vi "SetHasckelAO.vi"(0 "FPGA API in":refnum<class "FPGA API Mock.lvclass">, 5 "Haskel in":dbl, 11 "error in (no error)":errorcluster) -> (4 "FPGA API out":refnum<class "FPGA API Mock.lvclass">, 15 "error out":errorcluster)   [LabVIEW 2019, in "FPGA API Mock.lvclass"]
uses:
  FPGA API Mock.lvclass
  FPGA API Mock.lvclass/FPGA API Mock.ctl
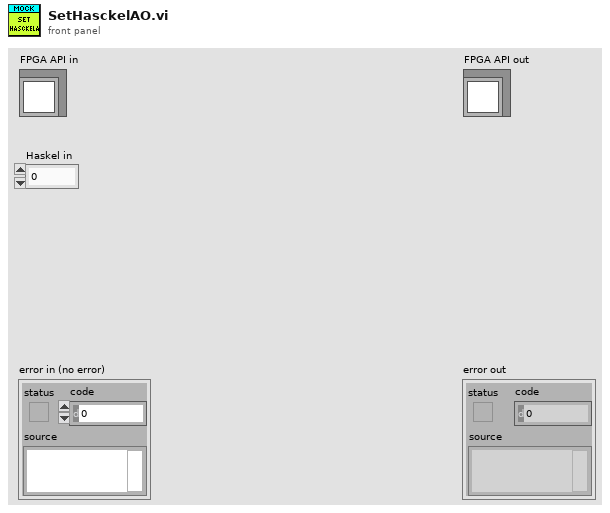
[diagram p1: front panel]
types:
  T1 = typedef "FPGA API Mock.lvclass/Data.ctl" = cluster{"DO":bool[], "DI":bool[], "AI":dbl[], "AO":dbl[]}
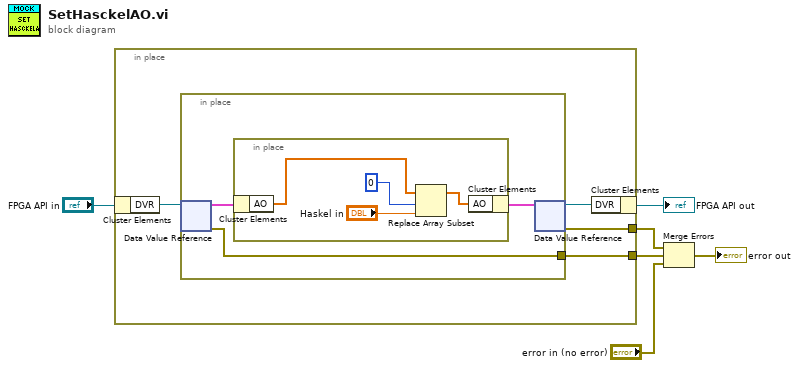
[diagram p0: block diagram]
diagram:
  n1 = in-place {
    in-place-border: [w8] -> w2
    in-place-border: [w7] -> w1
    n2 = in-place-cluster #1("FPGA API in") -> ("DVR"=w9:refnum<data-value>)
    n3 = in-place {
      in-place-border: [w11] -> w8
      n4 = in-place-dvr #2(w9) -> (w13:T1, w11:errorcluster)
      n5 = in-place {
        n6 = in-place-cluster #3(w13) -> ("AO"=w17:dbl[])
        n7 = Replace Array Subset(array=w17, new element="Haskel in", index=0) -> (w16:dbl[])
        n8 = in-place-cluster #3("AO"=w16) -> (w12:T1)
      }
      n9 = in-place-dvr #2(w12) -> (w10:refnum<data-value>, w7:errorcluster)
    }
    n10 = in-place-cluster #1("DVR"=w10) -> (→"FPGA API out":refnum<class "FPGA API Mock.lvclass">)
  }
  n11 = Merge Errors(w1, w2, "error in (no error)") -> (→"error out":errorcluster)
